vi "checkBeginEnemyPossessionAtEnemyFieldPlay.vi"(8 "error in (no error)":errorcluster, 10 "Game":refnum<class "Game.lvclass">, 11 "EnemyPossessionAtEnemyFieldPlay in":refnum<class "EnemyPossessionAtEnemyFieldPlay.lvclass">) -> (0 "error out":errorcluster, 2 "Begin?":bool, 3 "EnemyPossessionAtEnemyFieldPlay out":refnum<class "EnemyPossessionAtEnemyFieldPlay.lvclass">)   [LabVIEW 2023, in "EnemyPossessionAtEnemyFieldPlay.lvclass"]
uses:
  EnemyPossessionAtEnemyFieldPlay.lvclass
  Game_class/Game.lvclass
  Game_class/Game.lvclass/Game.ctl
  Events_class/Events.lvclass/Events.ctl
  Object_class/Object.lvclass/Object.ctl
  Game_class/Read Referee.vi
  Game_class/Read EventsRef.vi
  Game_class/Read BallRef.vi
  Object_class/Read x.vi
  Events_class/Read enemy_ball_possesion.vi
  Ball_class/Ball.lvclass
  Referee_class/Referee.lvclass
  Events_class/Events.lvclass
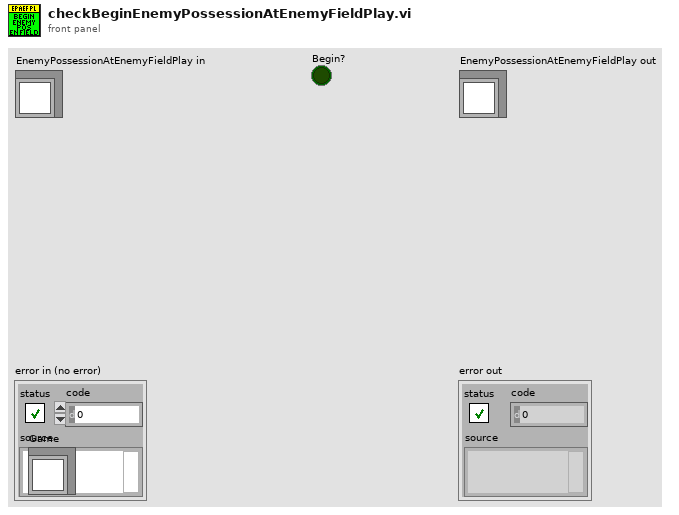
[diagram p1: front panel]
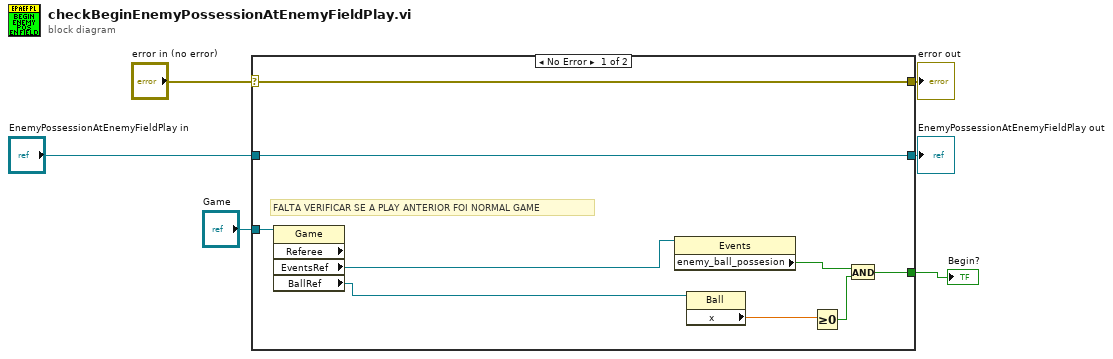
[diagram p0: block diagram]
diagram:
  n1 = case shown="No Error" "error in (no error)" {
    selector: "error in (no error)" -> [w14 w17]
    tunnel: [w14 w17] -> w5
    tunnel: [w15 w16] -> w3
    tunnel: "EnemyPossessionAtEnemyFieldPlay in" -> [w15 w16]
    tunnel: "Game" -> [w13 _]
    tunnel: [w8 _] -> w1
    frame No Error {
      # "FALTA VERIFICAR SE A PLAY ANTERIOR FOI NORMAL GAME"
      n2 = property class="Game" props=["Referee", "EventsRef", "BallRef"](reference=w13) -> ("EventsRef"=w12:refnum<class "Events.lvclass">, "BallRef"=w11:refnum<class "Ball.lvclass">)  [unwired: 1 in, 3 out]
      n3 = property class="Events"(reference=w12) -> ("enemy_ball_possesion"=w7:bool)  [unwired: 1 in, 2 out]
      n4 = property class="Ball"(reference=w11) -> ("x"=w10:dbl)  [unwired: 1 in, 2 out]
      n5 = Greater Or Equal To 0?(x=w10) -> (x >= 0?=w9:bool)
      n6 = And(x=w7, y=w9) -> (x .and. y?=w8:bool)
    }
    frame Error {
    }
  }
  "error out" <- w5
  "EnemyPossessionAtEnemyFieldPlay out" <- w3
  "Begin?" <- w1
